vi "Read ECAT VARs.vi"(7 "R/W Case":T7, 8 "error in (no error)":errorcluster, 9 "Output FIFO buffer in":dbl[](array[numeric]), 10 "I/O Input Data in":T1 {"BD Refs"."Data Reference" format="%.0x"}, 11 "I/O Output Vars in":T4[](array[typedef]) {"VS ref" format="%.0x"}) -> (0 "error out":errorcluster, 1 "Output FIFO buffer out":dbl[](array[numeric]), 2 "I/O Input Data out":T1 {"BD Refs"."Data Reference" format="%.0x"}, 3 "I/O Output Vars out":T4[](array[typedef]) {"VS ref" format="%.0x"})   [LabVIEW 2015, in "Scan Engine Custom Device.lvlib"]
uses:
  Type Defs/RW Case.ctl
  Type Defs/Generic ECAT Slave IOV Cluster.ctl
  <vilib>/NI Veristand/Custom Device API/Custom Device Item Ref.ctl
  Type Defs/UDV Data Type.ctl
  Type Defs/Input Data.ctl
  <vilib>/NI Veristand/Custom Device API/Block Data Reference.ctl
  <vilib>/NI Veristand/Custom Device API/Data Reference.ctl
  <vilib>/NI Veristand/Custom Device API/Global Data Refs.vi
  Scan Engine Custom Device.lvlib
  <vilib>/NI Veristand/Custom Device API/Custom Device API.lvlib
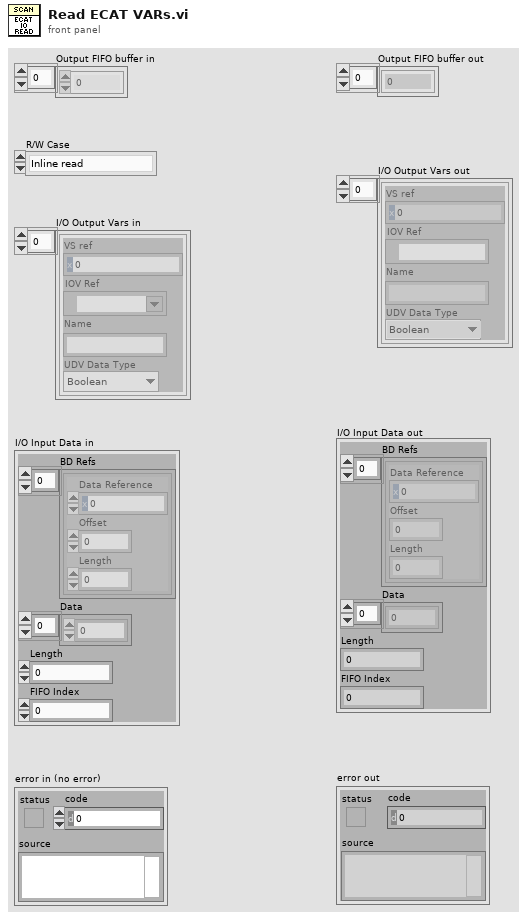
[diagram p1: front panel]
types:
  T1 = typedef "Scan Engine Custom Device.lvlib/Input Data.ctl" = cluster{"BD Refs":T2[], "Data":dbl[], "Length":i32, "FIFO Index":i32}
  T2 = typedef "Custom Device API.lvlib/Block Data Reference.ctl" = cluster{"Data Reference":T3, "Offset":u64, "Length":u64}
  T3 = typedef "Custom Device API.lvlib/Data Reference.ctl" = i32
  T4 = typedef "Scan Engine Custom Device.lvlib/Generic ECAT Slave IOV Cluster.ctl" = cluster{"VS ref":T5, "IOV Ref":refnum<k21>, "Name":string, "UDV Data Type":T6}
  T5 = typedef "Custom Device API.lvlib/Custom Device Item Ref.ctl" = u64
  T6 = typedef "Scan Engine Custom Device.lvlib/UDV Data Type.ctl" = enum16{"Boolean", "Fixed Point", "Int8", "Int16", "Int32", "Int64", "U32 Bit Field", "UInt8", "UInt16", "UInt32", "UInt64", "Other"}
  T7 = typedef "Scan Engine Custom Device.lvlib/RW Case.ctl" = enum16{"Inline read", "Inline write", "Async - Inline loop read", "Async - Inline loop write", "Async loop (read/write)"}
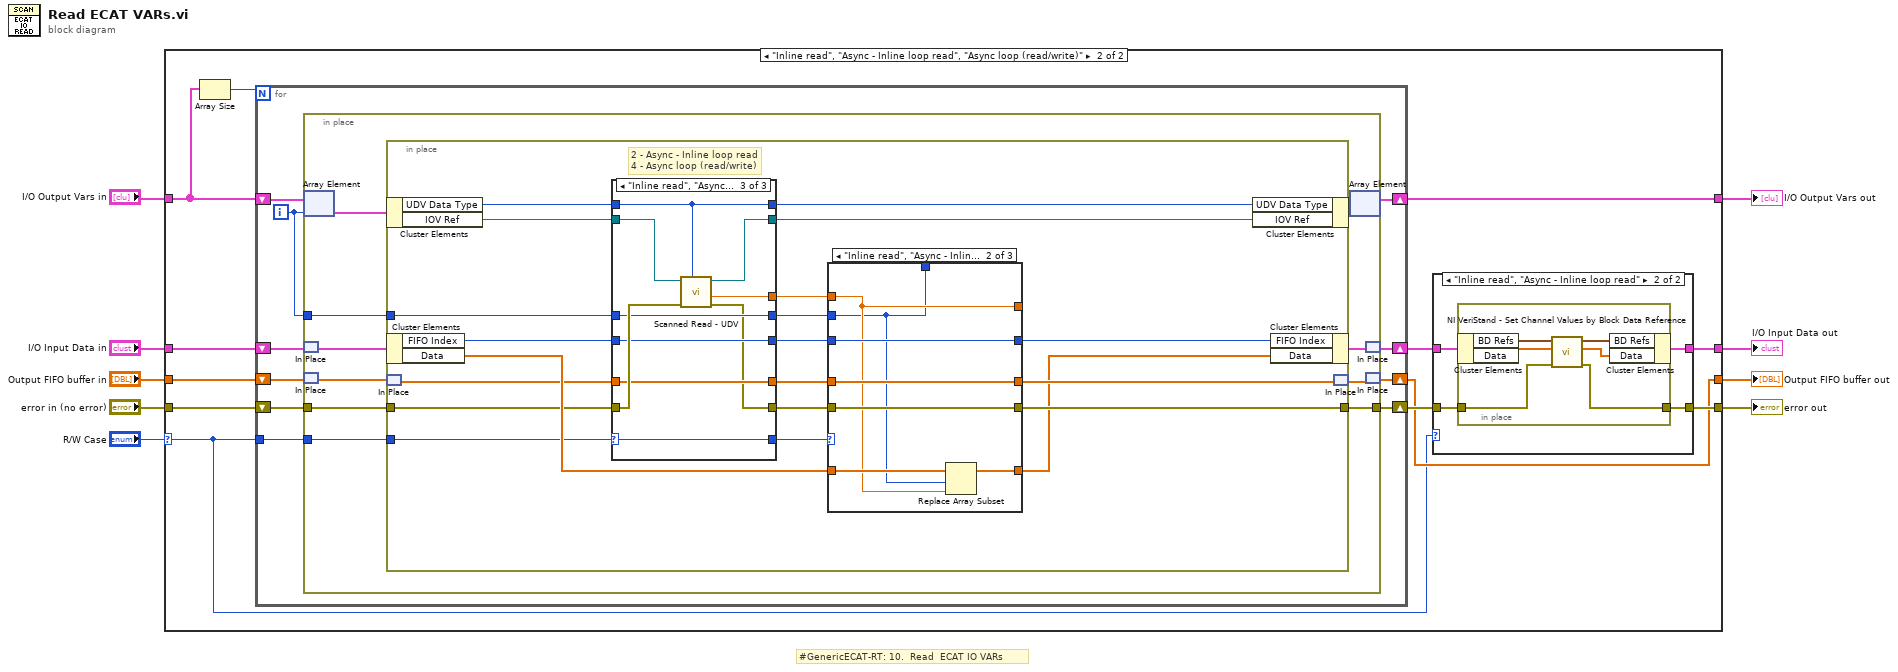
[diagram p0: block diagram]
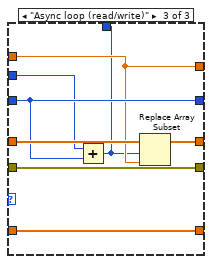
[diagram p5: hidden frame]
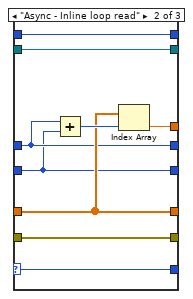
[diagram p7: hidden frame]
diagram:
  # "#GenericECAT-RT: 10.  Read  ECAT IO VARs"
  n1 = case shown="\"Inline read\", \"Async - Inline loop read\", \"Async loop (read/write)\"" "R/W Case" {
    selector: "R/W Case" -> [_ w14]
    tunnel: [w11 w15] -> w9
    tunnel: "Output FIFO buffer in" -> [w11 w25]
    tunnel: [w12 w18] -> w1
    tunnel: [w13 w24] -> w3
    tunnel: "I/O Input Data in" -> [w12 w23]
    tunnel: "I/O Output Vars in" -> [w13 w22]
    tunnel: [w10 w17] -> w7
    tunnel: "error in (no error)" -> [w10 w20]
    frame Default {
    }
    frame "Inline read", "Async - Inline loop read", "Async loop (read/write)" {
      n2 = Array Size(array=w22) -> (size(s)=w21:i32)
      n3 = for {
        N: w21 -> [_]
        shift-right: [w46] -> w24
        shift-left: w22 -> [w47]
        shift-right: [w38] -> w16
        shift-left: w23 -> [w41]
        shift-right: [w44] -> w15
        shift-left: w25 -> [w45]
        shift-right: [w42] -> w19
        shift-left: w20 -> [w43]
        tunnel: w14 -> [w40]
        i -> [w39]
        n4 = in-place {
          in-place-border: w43 -> [w54]
          in-place-border: [w48] -> w42
          in-place-border: w40 -> [w53]
          in-place-border: w39 -> [w52]
          n5 = in-place-array #1(w47, w39) -> (w57:T4)
          n6 = in-place-match #2(w41) -> (w56:T1)
          n7 = in-place-match #3(w45) -> (w55:dbl[])
          n8 = in-place {
            in-place-border: w54 -> [w70]
            in-place-border: w53 -> [w75]
            in-place-border: w52 -> [w71]
            in-place-border: [w68] -> w48
            # "2 - Async - Inline loop read\n4 - Async loop (read/write)"
            n9 = in-place-cluster #4(w57) -> ("UDV Data Type"=w74:T6, "IOV Ref"=w73:refnum<k21>)
            n10 = in-place-cluster #5(w56) -> ("FIFO Index"=w77:i32, "Data"=w76:dbl[])
            n11 = in-place-match #6(w55) -> (w72:dbl[])
            n12 = case shown="\"Inline read\", \"Async loop (read/write)\"" w75 {
              selector: w75 -> [w99 w109 w116]
              tunnel: w74 -> [w100 w107 w117]
              tunnel: w73 -> [w101 w108 w124]
              tunnel: w77 -> [w103 w110 w120]
              tunnel: w72 -> [w104 w113 w119]
              tunnel: [w104 w113 w119] -> w63
              tunnel: w71 -> [w102 w111 w121]
              tunnel: [_ w112 w115] -> w61
              tunnel: [w102 w111 w121] -> w65
              tunnel: [w103 w110 w120] -> w64
              tunnel: [w99 w109 w116] -> w58
              tunnel: [w101 w108 w123] -> w60
              tunnel: [w100 w107 w117] -> w69
              tunnel: w70 -> [w105 w106 w122]
              tunnel: [w105 w106 w118] -> w62
              frame Default {
              }
              frame "Async - Inline loop read" {
                n13 = Add(x=w111, y=w110) -> (x+y=w114:i32)
                n14 = Index Array(array=w113, index=w114) -> (element=w112:dbl)
              }
              frame "Inline read", "Async loop (read/write)" {
                n15 = call "Scanned Read - UDV.vi"("UDV Data Type"=w117, "error in (no error)"=w122, "IOV ref in"=w124) -> ("error out"=w118:errorcluster, "data out"=w115:dbl, "IOV ref out"=w123:refnum<k21>)  [unwired: 6 in]
              }
            }
            n16 = case shown="\"Inline read\", \"Async - Inline loop read\"" w58 {
              tunnel: w65 -> [w79 w84 w92]
              tunnel: w64 -> [w83 w86 w94]
              tunnel: w61 -> [w78 w85 w93]
              tunnel: w63 -> [w80 w87 w98]
              tunnel: w62 -> [w81 w88 w96]
              tunnel: w76 -> [w82 w90 w95]
              tunnel: [w83 w86 w94] -> w67
              tunnel: [w82 w89 w95] -> w59
              tunnel: [w81 w88 w96] -> w68
              tunnel: [w80 w87 w97] -> w66
              tunnel: [w78 w85 w93] -> _
              tunnel: [w79 w84 w91] -> _
              frame Default {
              }
              frame "Inline read", "Async - Inline loop read" {
                n17 = Replace Array Subset(array=w90, new element=w85, index=w84) -> (w89:dbl[])
              }
              frame "Async loop (read/write)" {
                n18 = Add(x=w92, y=w94) -> (x+y=w91:i32)
                n19 = Replace Array Subset(array=w98, new element=w93, index=w91) -> (w97:dbl[])
              }
            }
            n20 = in-place-cluster #4("UDV Data Type"=w69, "IOV Ref"=w60) -> (w51:T4)
            n21 = in-place-cluster #5("FIFO Index"=w67, "Data"=w59) -> (w50:T1)
            n22 = in-place-match #6(w66) -> (w49:dbl[])
          }
          n23 = in-place-array #1(w51) -> (w46:T4[])  [unwired: 1 out]
          n24 = in-place-match #2(w50) -> (w38:T1)
          n25 = in-place-match #3(w49) -> (w44:dbl[])
        }
      }
      n26 = case shown="\"Inline read\", \"Async - Inline loop read\"" w14 {
        tunnel: w16 -> [w26 w28]
        tunnel: w19 -> [w27 w31]
        tunnel: [w27 w30] -> w17
        tunnel: [w26 w29] -> w18
        frame Default {
        }
        frame "Inline read", "Async - Inline loop read" {
          n27 = in-place {
            in-place-border: w31 -> [w35]
            in-place-border: [w34] -> w30
            n28 = in-place-cluster #7(w28) -> ("BD Refs"=w32:T2[], "Data"=w33:dbl[])
            n29 = call <vilib>:"NI VeriStand - Set Channel Values by Block Data Reference.vi"("error in (no error)"=w35, "Values Array in"=w33, "Block Data Ref"=w32) -> ("error out"=w34:errorcluster, "Values Array out"=w36:dbl[], "Block Data Ref dup"=w37:T2[])  [unwired: 6 in]
            n30 = in-place-cluster #7("BD Refs"=w37, "Data"=w36) -> (w29:T1)
          }
        }
      }
    }
  }
  "Output FIFO buffer out" <- w9
  "error out" <- w7
  "I/O Output Vars out" <- w3
  "I/O Input Data out" <- w1
